vi "Main.vi"() -> ()   [LabVIEW 2015]
doc: "This template is for the Queued Message Handler design pattern.\n\nThe Event Handling Loop generates messages based on user interface actions.\n\nThe Message Handling Loop processes messages generated by the Event Handling Loop, or by other messages. The messages are string values, so new messages can be added easily to the Message Cases case structure in the Message Handling Loop. Each message cluster can also provide an optional value for Message Data, which is a variant that can be converted to whatever message-specific data is required."
uses:
  controls/UI Data.ctl
  support/User Event - Stop/User Event - Stop.lvlib
  support/Message Queue/Message Queue.lvlib
  support/Boiler System Globals.vi
panel:
  out "Display <Replace Me>":string
  in  "Do Something Else <Replace Me>":bool
  in  "Do Something <Replace Me>":bool
  in  "Stop Button":bool
  # "These controls have associated \"Value Changed\" events configured in the Event Structure on the diagram.\n\nReplace them (and reconfigure the Event Structure) with the controls you need for your application."
  # "This template is for the Queued Message Handler design pattern.\n\nSee the block diagram for more information on how to use this template."
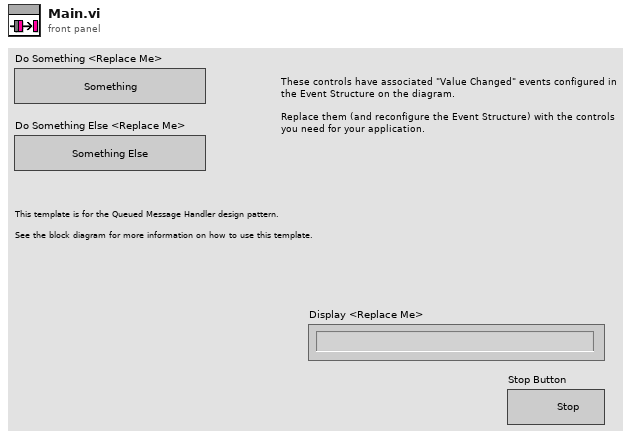
[diagram p1: front panel]
types:
  T1 = typedef "UI Data.ctl" = cluster{"Boolean <Replace Me>":bool, "String <Replace Me>":string, "Numeric <Replace Me>":dbl, "Do Something Ref":refnum<vi>, "Do Something Else Ref":refnum<vi>, "Data Display Ref":refnum<vi>, "Stop Button Ref":refnum<vi>}
  T2 = typedef "Notifires.ctl" = cluster{"Handshake":refnum<notifier>, "Flame level":T3, "Controller Exit":refnum<notifier>, "Boiler Exit":refnum<notifier>}
  T3 = typedef "Notifiers.ctl" = refnum<notifier>
  T4 = typedef "Message Queue.lvlib/All Message Queues.ctl" = cluster{"MHL":refnum<queue>, "Boiler Controller":refnum<queue>, "Boiler":refnum<queue>}
  T5 = enum32{"invalid app kind", "Development System", "Run Time System", "Student Edition", "Embedded LabVIEW", "Evaluation", "Custom"}
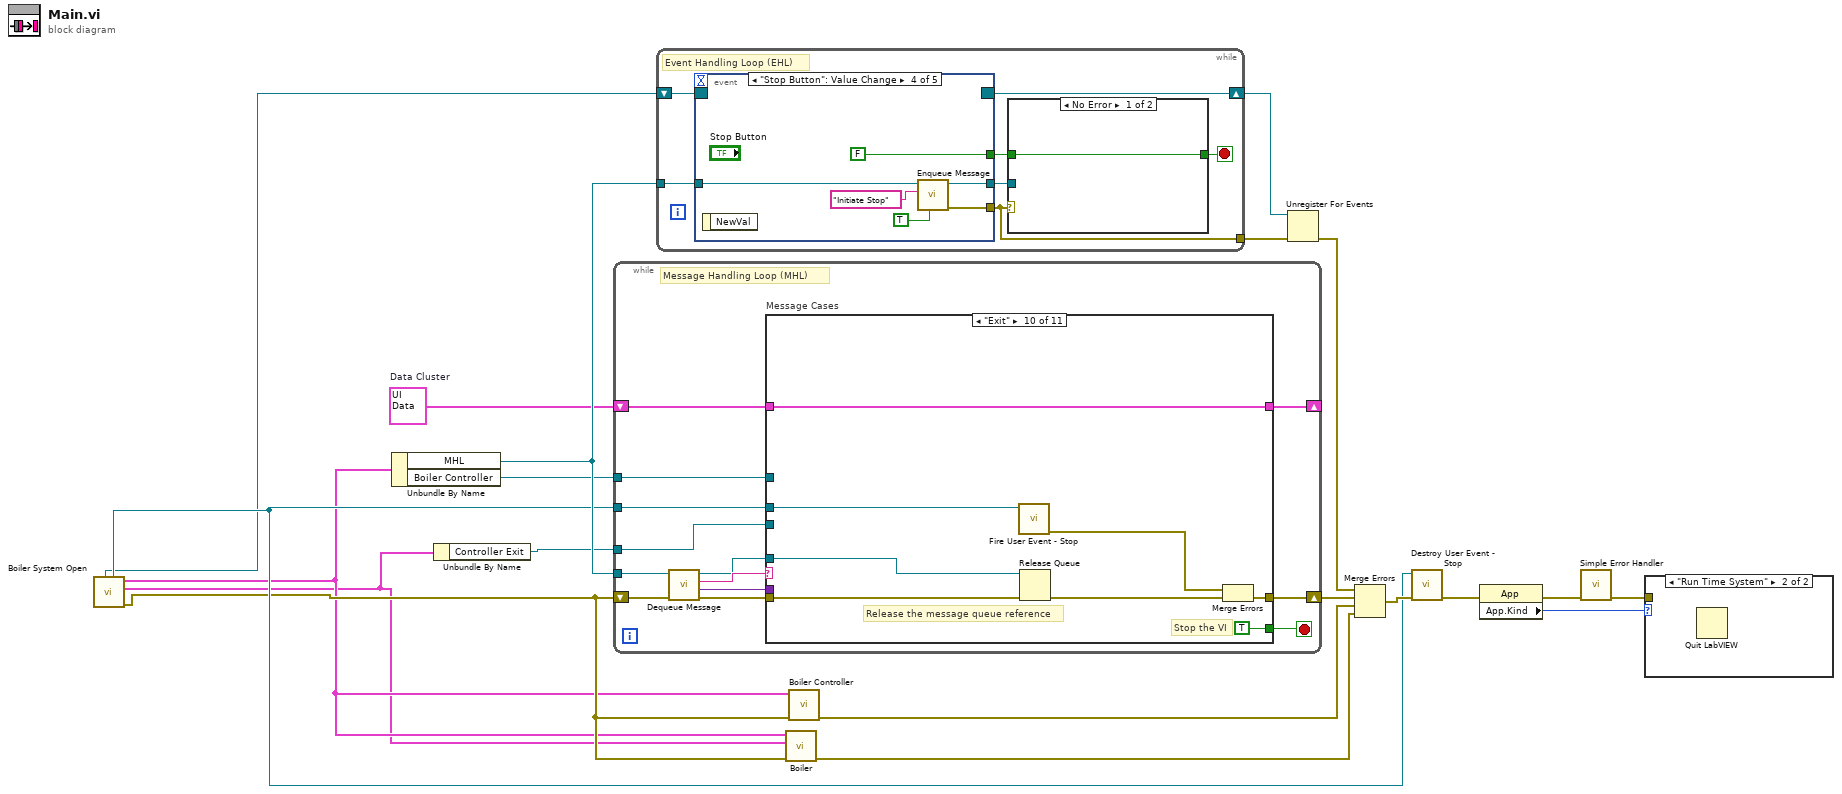
[diagram p0: block diagram]
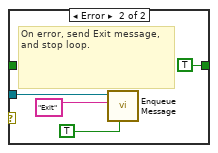
[diagram p3: hidden frame]
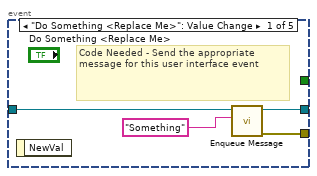
[diagram p4: hidden frame]
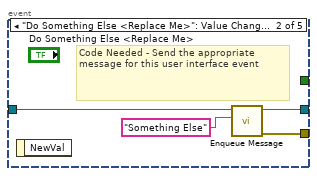
[diagram p5: hidden frame]
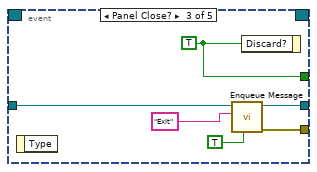
[diagram p6: hidden frame]
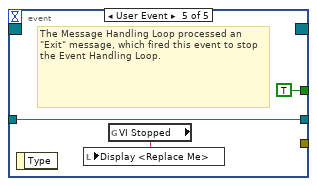
[diagram p7: hidden frame]
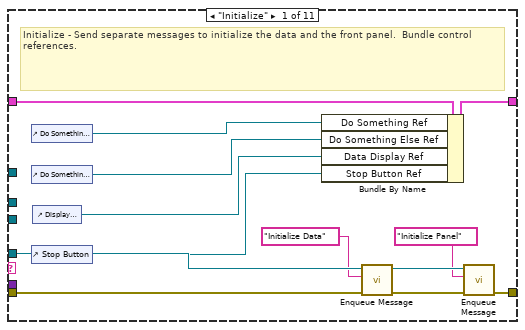
[diagram p8: hidden frame]
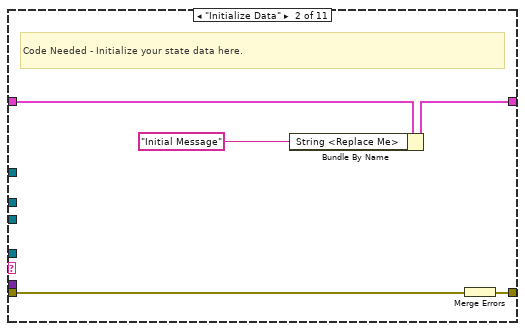
[diagram p9: hidden frame]
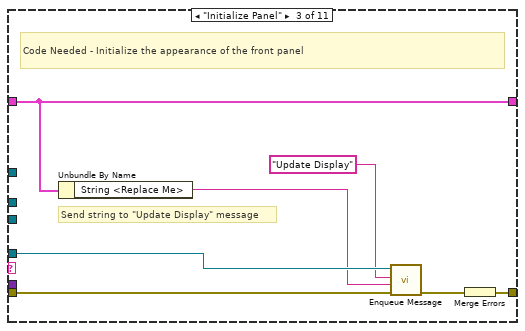
[diagram p10: hidden frame]
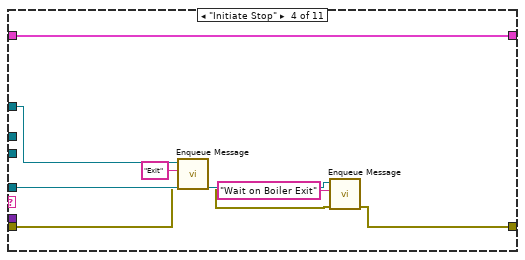
[diagram p11: hidden frame]
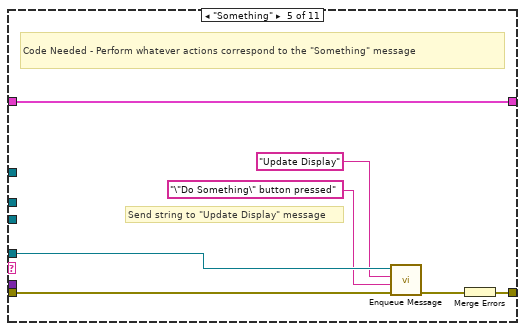
[diagram p12: hidden frame]
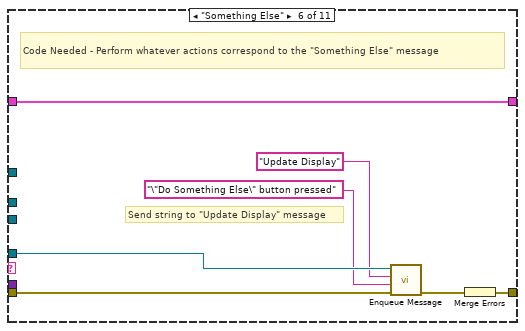
[diagram p13: hidden frame]
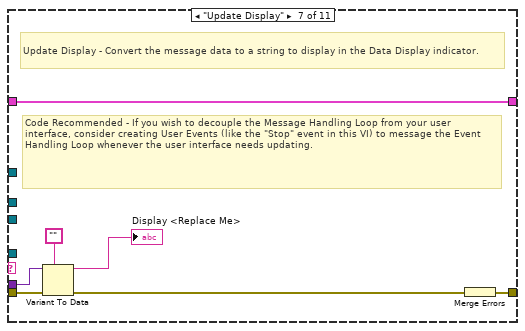
[diagram p14: hidden frame]
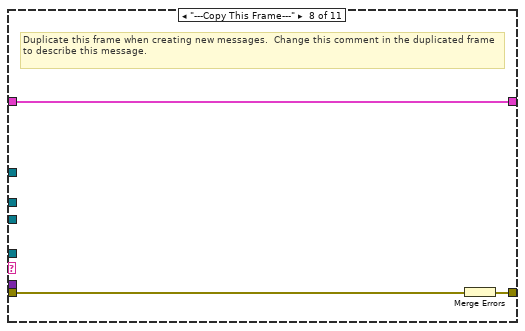
[diagram p15: hidden frame]
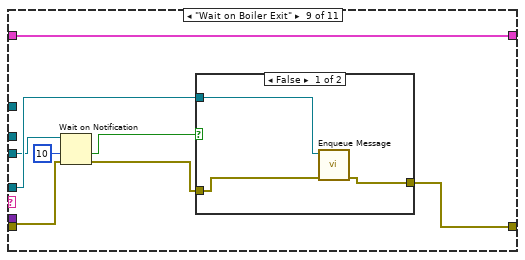
[diagram p16: hidden frame]
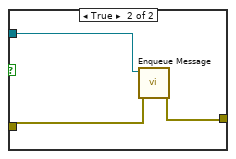
[diagram p17: hidden frame]
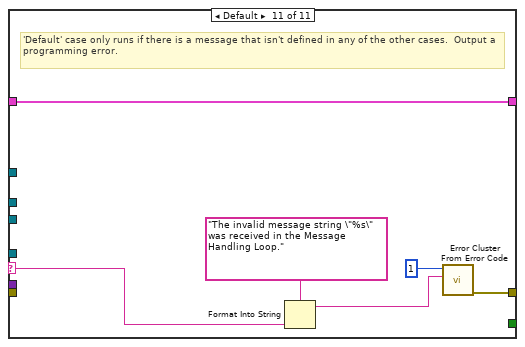
[diagram p18: hidden frame]
diagram:
  w13 = T1 {"Boolean <Replace Me>"=TRUE, "String <Replace Me>"="", "Numeric <Replace Me>"=0.0, "Do Something Ref"=refnum, "Do Something Else Ref"=refnum, "Data Display Ref"=refnum, "Stop Button Ref"=refnum}  # Data Cluster
  n1 = call "Boiler System Open.vi"() -> ("error out"=w5:errorcluster, "Notifiers"=w2:T2, "Message Queues out"=w3:T4, "User Event - Stop"=w7:refnum<user-event>, "Stop Event Registration Refnum"=w6:refnum<event-registration>)  [unwired: 7 in]
  n2 = Unbundle By Name(w3) -> ("MHL"=w19:refnum<queue>, "Boiler Controller"=w11:refnum<queue>)
  n3 = Unbundle By Name(w2) -> ("Controller Exit"=w1:refnum<notifier>)
  n4 = while {
    tunnel: w19 -> [w23]
    shift-right: [w32] -> _
    shift-left: w13 -> [w33]
    tunnel: w7 -> [w29]
    shift-right: [w30] -> w20
    shift-left: w5 -> [w28]
    tunnel: w11 -> [w22]
    tunnel: w1 -> [w21]
    stop <- w31 stop-if-true
    # "Message Handling Loop (MHL)"
    n5 = call "Dequeue Message.vi"("error in (no error)"=w28, "Message Queue"=w23) -> ("error out"=w27:errorcluster, "Message Data"=w25:variant, "Message"=w26:string, "dup Message Queue"=w24:refnum<queue>)  [unwired: 6 in]
    n6 = case "Message Cases" shown="\"Exit\"" w26 {
      selector: w26 -> [_ _ _ _ _ _ _ _ _ _ w116]
      tunnel: w24 -> [w42 _ w55 w64 w69 w76 _ _ w97 w112 _]
      tunnel: w27 -> [w45 w51 w56 w61 w71 w78 w85 w90 w94 w105 _]
      tunnel: [w46 w47 w57 w59 w72 w79 w86 w88 w96 w108 w114] -> w30
      tunnel: w33 -> [w39 w50 w58 w66 w73 w80 w87 w89 w98 w111 w118]
      tunnel: [w38 w49 w58 w66 w73 w80 w87 w89 w98 w111 w118] -> w32
      tunnel: [_ _ _ _ _ _ _ _ _ TRUE _] -> w31
      tunnel: w25 -> [_ _ _ _ _ _ w84 _ _ _ _]
      tunnel: w29 -> [_ _ _ _ _ _ _ _ _ w107 _]
      tunnel: w22 -> [_ _ _ w65 _ _ _ _ _ _ _]
      tunnel: w21 -> [_ _ _ _ _ _ _ _ w91 _ _]
      frame "Initialize" {
        # "Initialize - Send separate messages to initialize the data and the front panel.  Bundle control references."
        n7 = control-ref of="Do Something <Replace Me>"() -> (w37:refnum<vi>)
        n8 = control-ref of="Do Something Else <Replace Me>"() -> (w36:refnum<vi>)
        n9 = control-ref of="Stop Button"() -> (w34:refnum<vi>)
        n10 = control-ref of="Display <Replace Me>"() -> (w35:refnum<vi>)
        n11 = Bundle By Name(cluster=w39, "Do Something Ref"=w37, "Do Something Else Ref"=w36, "Data Display Ref"=w35, "Stop Button Ref"=w34) -> (w38:T1)
        n12 = call "Enqueue Message.vi"("error in (no error)"=w45, "Message"="Initialize Data", "Message Queue"=w42) -> ("error out"=w44:errorcluster, "dup Message Queue"=w43:refnum<queue>)  [unwired: 7 in]
        n13 = call "Enqueue Message.vi"("error in (no error)"=w44, "Message"="Initialize Panel", "Message Queue"=w43) -> ("error out"=w46:errorcluster)  [unwired: 7 in, 1 out]
      }
      frame "Initialize Data" {
        # "Code Needed - Initialize your state data here."
        n14 = Bundle By Name(cluster=w50, "String <Replace Me>"="Initial Message" ("Initial Message")) -> (w49:T1)
        n15 = Merge Errors(w51) -> (w47:errorcluster)
      }
      frame "Initialize Panel" {
        # "Send string to \"Update Display\" message"
        # "Code Needed - Initialize the appearance of the front panel"
        n16 = Unbundle By Name(w58) -> ("String <Replace Me>"=w52:string)
        n17 = call "Enqueue Message.vi"("error in (no error)"=w56, "Message Data"=w52, "Message"="Update Display", "Message Queue"=w55) -> ("error out"=w54:errorcluster)  [unwired: 6 in, 1 out]
        n18 = Merge Errors(w54) -> (w57:errorcluster)
      }
      frame "Initiate Stop" {
        n19 = call "Enqueue Message.vi"("error in (no error)"=w61, "Message"="Exit", "Message Queue"=w65) -> ("error out"=w60:errorcluster)  [unwired: 7 in, 1 out]
        n20 = call "Enqueue Message.vi"("error in (no error)"=w60, "Message"="Wait on Boiler Exit", "Message Queue"=w64) -> ("error out"=w59:errorcluster)  [unwired: 7 in, 1 out]
      }
      frame "Something" {
        # "Send string to \"Update Display\" message"
        # "Code Needed - Perform whatever actions correspond to the \"Something\" message"
        n21 = call "Enqueue Message.vi"("error in (no error)"=w71, "Message Data"="\"Do Something\" button pressed" ("\"Do Something\" button pressed"), "Message"="Update Display", "Message Queue"=w69) -> ("error out"=w70:errorcluster)  [unwired: 6 in, 1 out]
        n22 = Merge Errors(w70) -> (w72:errorcluster)
      }
      frame "Something Else" {
        # "Send string to \"Update Display\" message"
        # "Code Needed - Perform whatever actions correspond to the \"Something Else\" message"
        n23 = call "Enqueue Message.vi"("error in (no error)"=w78, "Message Data"="\"Do Something Else\" button pressed" ("\"Do Something Else\" button pressed"), "Message"="Update Display", "Message Queue"=w76) -> ("error out"=w77:errorcluster)  [unwired: 6 in, 1 out]
        n24 = Merge Errors(w77) -> (w79:errorcluster)
      }
      frame "Update Display" {
        # "Code Recommended - If you wish to decouple the Message Handling Loop from your user interface, consider creating User Events (like the \"Stop\" event in this VI) to message the Event Handling Loop whenever the user interface needs updating."
        # "Update Display - Convert the message data to a string to display in the Data Display indicator."
        n25 = Variant To Data(error in=w85, type="", Variant=w84) -> (data=→"Display <Replace Me>":string, error out=w82:errorcluster)
        n26 = Merge Errors(w82) -> (w86:errorcluster)
      }
      frame "---Copy This Frame---" {
        # "Duplicate this frame when creating new messages.  Change this comment in the duplicated frame to describe this message."
        n27 = Merge Errors(w90) -> (w88:errorcluster)
      }
      frame "Wait on Boiler Exit" {
        n28 = Wait on Notification(notifier=w91, timeout in ms (-1)=10, error in (no error)=w94) -> (timed out?=w95:bool, error out=w93:errorcluster)  [unwired: 1 in, 2 out]
        n29 = case shown="False" w95 {
          tunnel: w97 -> [w101 w104]
          tunnel: w93 -> [w100 w103]
          tunnel: [w99 w102] -> w96
          frame False {
            n30 = call "Enqueue Message.vi"("error in (no error)"=w100, "Message Queue"=w101) -> ("error out"=w99:errorcluster)  [unwired: 8 in, 1 out]
          }
          frame True {
            n31 = call "Enqueue Message.vi"("error in (no error)"=w103, "Message Queue"=w104) -> ("error out"=w102:errorcluster)  [unwired: 8 in, 1 out]
          }
        }
      }
      frame "Exit" {
        # "Stop the VI"
        # "Release the message queue reference"
        n32 = call "Fire User Event - Stop.vi"("User Event - Stop"=w107) -> ("error out"=w106:errorcluster)  [unwired: 10 in]
        n33 = Release Queue(queue=w112, error in (no error)=w105) -> (error out=w109:errorcluster)  [unwired: 1 in, 2 out]
        n34 = Merge Errors(w106, w109) -> (w108:errorcluster)
      }
      frame Default {
        # "'Default' case only runs if there is a message that isn't defined in any of the other cases.  Output a programming error."
        n35 = Format Into String(format string="The invalid message string \"%s\" was received in the Message Handling Loop." ("Unknown Message Error Text"), w116) -> (resulting string=w113:string)  [unwired: 2 in, 1 out]
        n36 = call <vilib>:"Error Cluster From Error Code.vi"("error message (\"\")"=w113, "error code (0)"=1) -> ("error out"=w114:errorcluster)  [unwired: 7 in]
      }
    }
  }
  n37 = while {
    tunnel: w19 -> [w125]
    tunnel: [w121] -> w15
    shift-right: [w119] -> w14
    shift-left: w6 -> [w120]
    stop <- w123 stop-if-true
    # "Event Handling Loop (EHL)"
    n38 = event shown="[3] \"Stop Button\": Value Change" {
      selector: w120 -> [_ _ _ _ _]
      dyn-events: [_ _ _ _ _] -> w119
      timeout: _ -> [_ _ _ _ _]
      tunnel: [_ _ w144 FALSE ("Discard?") TRUE ("Discard?")] -> w124
      tunnel: w125 -> [w134 w138 w143 w150 w153]
      tunnel: [w133 w136 w142 w149 _] -> w121
      tunnel: [w132 w137 w141 w147 w153] -> w122
      event "Do Something <Replace Me>": Value Change {
        # "Code Needed - Send the appropriate message for this user interface event"
        n39 = event-data() -> ()  [unwired: 1 in, 1 out]
        n40 = call "Enqueue Message.vi"("Message"="Something", "Message Queue"=w134) -> ("error out"=w133:errorcluster, "dup Message Queue"=w132:refnum<queue>)  [unwired: 8 in]
      }
      event "Do Something Else <Replace Me>": Value Change {
        # "Code Needed - Send the appropriate message for this user interface event"
        n41 = event-data() -> ()  [unwired: 1 in, 1 out]
        n42 = call "Enqueue Message.vi"("Message"="Something Else", "Message Queue"=w138) -> ("error out"=w136:errorcluster, "dup Message Queue"=w137:refnum<queue>)  [unwired: 8 in]
      }
      event Panel Close? {
        w144 = TRUE ("Discard?")
        n43 = event-data() -> ()  [unwired: 1 in, 1 out]
        n44 = call "Enqueue Message.vi"("Priority Message? (F)"=TRUE, "Message"="Exit", "Message Queue"=w143) -> ("error out"=w142:errorcluster, "dup Message Queue"=w141:refnum<queue>)  [unwired: 7 in]
        n45 = event-data("Discard?"=w144) -> ()  [unwired: 1 in, 1 out]
      }
      event "Stop Button": Value Change {
        n46 = event-data() -> ()  [unwired: 1 in, 1 out]
        n47 = call "Enqueue Message.vi"("Priority Message? (F)"=TRUE, "Message"="Initiate Stop", "Message Queue"=w150) -> ("error out"=w149:errorcluster, "dup Message Queue"=w147:refnum<queue>)  [unwired: 7 in]
      }
      event User Event {
        # "The Message Handling Loop processed an \"Exit\" message, which fired this event to stop the Event Handling Loop."
        n48 = event-data() -> ()  [unwired: 1 in, 1 out]
        n49 = global read "Boiler System Globals.vi" "VI Stopped"() -> (w151:string)
        n50 = local write "Display <Replace Me>"(w151) -> ()
      }
    }
    n51 = case shown="No Error" w121 {
      tunnel: [w126 TRUE ("Discard?")] -> w123
      tunnel: w124 -> [w126 _]
      tunnel: w122 -> [_ w129]
      frame No Error {
      }
      frame Error {
        # "On error, send Exit message, and stop loop."
        n52 = call "Enqueue Message.vi"("Priority Message? (F)"=TRUE, "Message"="Exit", "Message Queue"=w129) -> ()  [unwired: 7 in, 2 out]
      }
    }
  }
  n53 = call "Boiler.vi"("error in"=w5, "Notifiers"=w2, "Message Queues"=w3) -> ("error out"=w4:errorcluster)  [unwired: 8 in]
  n54 = call "Boiler Controller.vi"("error in"=w5, "Message Queues"=w3) -> ("error out"=w12:errorcluster)  [unwired: 9 in]
  n55 = Unregister For Events(event registration refnum=w14, error in=w15) -> (error out=w16:errorcluster)
  n56 = Merge Errors(w16, w20, w12, w4) -> (w17:errorcluster)
  n57 = call "Destroy User Event - Stop.vi"("error in (no error)"=w17, "User Event - Stop"=w7) -> ("error out"=w18:errorcluster)  [unwired: 9 in]
  n58 = property class="App"(error in=w18) -> (error out=w10:errorcluster, "App.Kind"=w9:T5)  [unwired: 1 in, 1 out]
  n59 = call <vilib>:"Simple Error Handler.vi"("error in (no error)"=w10) -> ("error out"=w8:errorcluster)  [unwired: 4 in, 4 out]
  n60 = case shown="\"Run Time System\"" w9 {
    tunnel: w8 -> [_ _]
    frame Default {
    }
    frame "Run Time System" {
      n61 = Quit LabVIEW() -> ()  [unwired: 1 in]
    }
  }
